vi "Capture@FeatureMatchOne__Parameter.vi"(1 "ParamterIn":string) -> (0 "ParamterOut":string)   [LabVIEW 2020]
uses:
  MainFrame/Global.vi
panel:
  out "Image":T1(plugin-control)
  in  "Picture":string(combo)
  in  "AngleEnd":string(combo)
  in  "AngleStart":string(combo)
  in  "Score":string(combo)="50"
  in  "Point":string(combo)
  in  "CamName":string(combo)
  in  "Confirm":bool
  # "Capture@FeatureMatchOne $Capture,$Picture,$Score,$Point(,$Angle=XX~XX)"
  # "Angle="
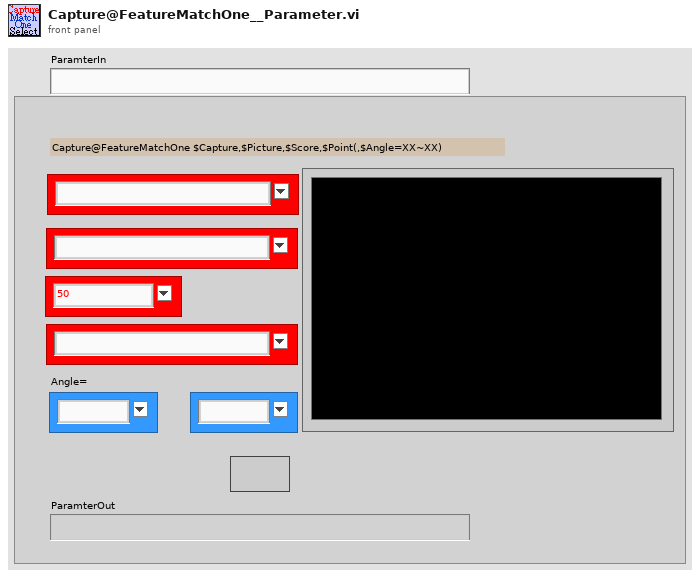
[diagram p1: front panel]
types:
  T1 = typedef "IMAQ Image.ctl" = refnum<image>
  T2 = enum16{"Get", "UpdatePointS", "Init", "UpdateIndex", "GetCurrent&Index+1", "GetWithIndex", "ChkLast", "GetCurrent"}
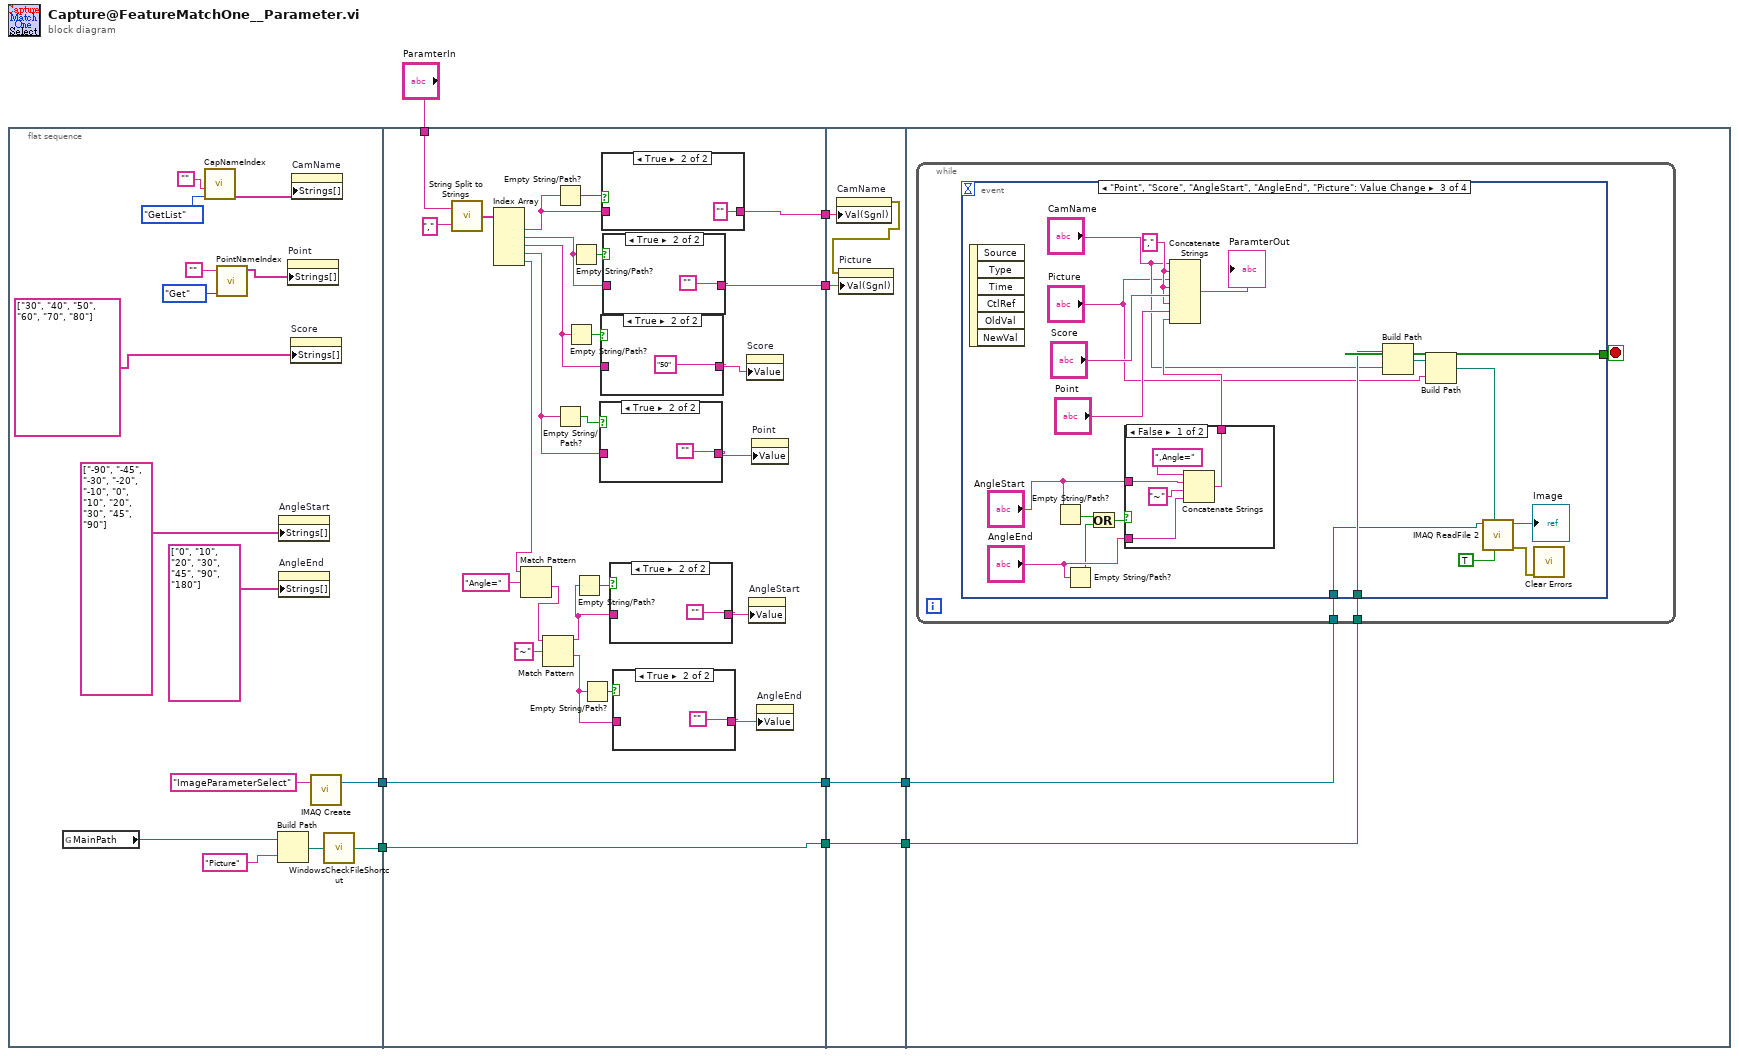
[diagram p0: block diagram]
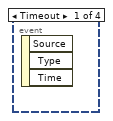
[diagram p8: hidden frame]
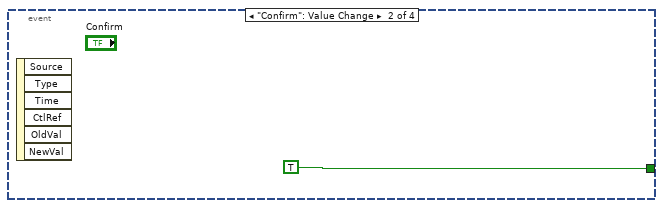
[diagram p9: hidden frame]
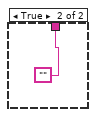
[diagram p10: hidden frame]
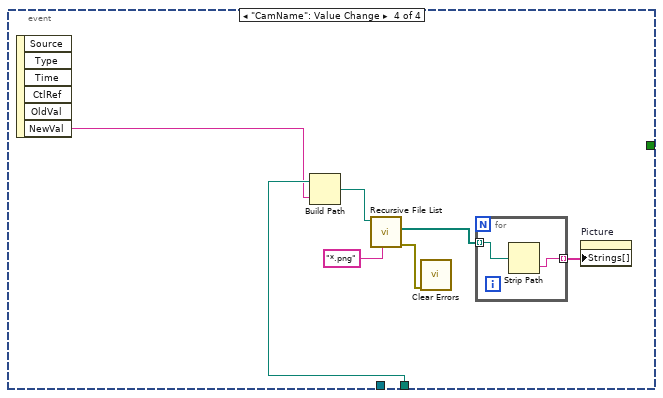
[diagram p11: hidden frame]
diagram:
  n1 = flat-sequence {
    tunnel: [w16] -> w8
    tunnel: [w10] -> w3
    tunnel: "ParamterIn" -> [w49]
    tunnel: w8 -> [w30]
    tunnel: [w30] -> w7
    tunnel: [w28] -> w4
    tunnel: w3 -> [w28]
    tunnel: [w26] -> w2
    tunnel: [w25] -> w1
    tunnel: w7 -> [w68]
    tunnel: [w68] -> w6
    tunnel: [w67] -> w5
    tunnel: w4 -> [w67]
    tunnel: w2 -> [w66]
    tunnel: w1 -> [w65]
    tunnel: w6 -> [w70]
    tunnel: w5 -> [w69]
    frame #0 {
      n2 = global read "Global.vi" "MainPath"() -> (w13:path)
      n3 = call "CapNameIndex.vi"("OP"=enum16{"AddCam", "GetIndex", "Init", "GetList"}."GetList", "CamName"="") -> ("DeviceList"=w23:string[])  [unwired: 2 in, 3 out]
      n4 = call "PointNameIndex.vi"("OP"=T2."Get", "PointName"="") -> ("PointNameList"=w19:string[])  [unwired: 4 in, 5 out]
      n5 = Build Path(base path=w13, name or relative path="Picture") -> (appended path=w11:path)
      n6 = property on="AngleStart" class="CmbBox"("Strings[]"=string[] ["-90", "-45", "-30", "-20", "-10", "0", "10", "20", "30", "45", "90"] ("Strings []")) -> ()  [unwired: 2 in, 2 out]
      n7 = property on="AngleEnd" class="CmbBox"("Strings[]"=string[] ["0", "10", "20", "30", "45", "90", "180"] ("Strings []")) -> ()  [unwired: 2 in, 2 out]
      n8 = property on="Point" class="CmbBox"("Strings[]"=w19) -> ()  [unwired: 2 in, 2 out]
      n9 = property on="Score" class="CmbBox"("Strings[]"=string[] ["30", "40", "50", "60", "70", "80"] ("Strings []")) -> ()  [unwired: 2 in, 2 out]
      n10 = property on="CamName" class="CmbBox"("Strings[]"=w23) -> ()  [unwired: 2 in, 2 out]
      n11 = call "IMAQ Create"("Image Name"="ImageParameterSelect") -> ("New Image"=w16:T1)  [unwired: 4 in, 1 out]
      n12 = call "WindowsCheckFileShortcut.vi"("LinkPath"=w11) -> ("TargetPath"=w10:path)  [unwired: 4 in]
    }
    frame #1 {
      n13 = call "String Split to Strings.vi"("search string/char (-)"=",", "String"=w49) -> ("Array"=w51:string[])
      n14 = Index Array(array=w51) -> (element #1=w29:string, element #2=w41:string, element #3=w44:string, element #4=w46:string, element #5=w40:string)  [unwired: 5 in]
      n15 = Match Pattern(string=w40, regular expression="Angle=") -> (after substring=w38:string)  [unwired: 1 in, 3 out]
      n16 = Match Pattern(string=w38, regular expression="~") -> (before substring=w35:string, after substring=w33:string)  [unwired: 1 in, 2 out]
      n17 = Empty String/Path?(string/path=w29) -> (empty?=w48:bool)
      n18 = Empty String/Path?(string/path=w46) -> (empty?=w47:bool)
      n19 = Empty String/Path?(string/path=w44) -> (empty?=w45:bool)
      n20 = Empty String/Path?(string/path=w41) -> (empty?=w42:bool)
      n21 = Empty String/Path?(string/path=w35) -> (empty?=w36:bool)
      n22 = Empty String/Path?(string/path=w33) -> (empty?=w34:bool)
      n23 = case shown="True" w47 {
        tunnel: [w60 ""] -> w27
        tunnel: w46 -> [w60 _]
        frame False {
        }
        frame True {
        }
      }
      n24 = case shown="True" w45 {
        tunnel: [w58 "50"] -> w43
        tunnel: w44 -> [w58 _]
        frame False {
        }
        frame True {
        }
      }
      n25 = case shown="True" w48 {
        tunnel: w29 -> [w62 _]
        tunnel: [w62 ""] -> w25
        frame False {
        }
        frame True {
        }
      }
      n26 = case shown="True" w42 {
        tunnel: [w56 ""] -> w26
        tunnel: w41 -> [w56 _]
        frame False {
        }
        frame True {
        }
      }
      n27 = case shown="True" w36 {
        tunnel: [w54 ""] -> w32
        tunnel: w35 -> [w54 _]
        frame False {
        }
        frame True {
        }
      }
      n28 = case shown="True" w34 {
        tunnel: [w52 ""] -> w31
        tunnel: w33 -> [w52 _]
        frame False {
        }
        frame True {
        }
      }
      n29 = property on="Score" class="CmbBox"("Value"=w43) -> ()  [unwired: 2 in, 2 out]
      n30 = property on="AngleStart" class="CmbBox"("Value"=w32) -> ()  [unwired: 2 in, 2 out]
      n31 = property on="Point" class="CmbBox"("Value"=w27) -> ()  [unwired: 2 in, 2 out]
      n32 = property on="AngleEnd" class="CmbBox"("Value"=w31) -> ()  [unwired: 2 in, 2 out]
    }
    frame #2 {
      n33 = property on="CamName" class="CmbBox"("Val(Sgnl)"=w65) -> (error out=w64:errorcluster)  [unwired: 2 in, 1 out]
      n34 = property on="Picture" class="CmbBox"(error in=w64, "Val(Sgnl)"=w66) -> ()  [unwired: 1 in, 2 out]
    }
    frame #3 {
      n35 = while {
        tunnel: w70 -> [w72]
        tunnel: w69 -> [w71]
        stop <- w73 stop-if-true
        n36 = event shown="[2] \"Point\", \"Score\", \"AngleStart\", \"AngleEnd\", \"Picture\": Value Change" {
          selector: _ -> [_ _ _ _]
          dyn-events: _ -> [_ _ _ _]
          timeout: _ -> [_ _ _ _]
          tunnel: [_ TRUE _ _] -> w73
          tunnel: w72 -> [_ _ w76 _]
          tunnel: w71 -> [_ _ w83 w103]
          event Timeout {
            n37 = event-data() -> ()  [unwired: 1 in, 3 out]
          }
          event "Confirm": Value Change {
            n38 = event-data() -> ()  [unwired: 1 in, 6 out]
          }
          event "Point", "Score", "AngleStart", "AngleEnd", "Picture": Value Change {
            w90 = "," ("string")
            n39 = event-data() -> ()  [unwired: 1 in, 6 out]
            n40 = Empty String/Path?(string/path="AngleStart") -> (empty?=w85:bool)
            n41 = Empty String/Path?(string/path="AngleEnd") -> (empty?=w84:bool)
            n42 = Or(x=w85, y=w84) -> (x .or. y?=w86:bool)
            n43 = case shown="False" w86 {
              tunnel: [w96 ""] -> w89
              tunnel: "AngleStart" -> [w95 _]
              tunnel: "AngleEnd" -> [w94 _]
              frame False {
                n44 = Concatenate Strings(",Angle=" ("string"), w95, "~", w94) -> (w96:string)
              }
              frame True {
              }
            }
            n45 = Concatenate Strings("CamName", w90, "Picture", w90, "Score", w90, "Point", w89) -> (→"ParamterOut":string)
            n46 = Build Path(base path=w83, name or relative path="CamName") -> (appended path=w81:path)
            n47 = Build Path(base path=w81, name or relative path="Picture") -> (appended path=w79:path)
            n48 = call "IMAQ ReadFile 2"("Use File Path Image Type"=TRUE, "File Path"=w79, "Image"=w76) -> ("error out"=w78:errorcluster, "Image Out"=→"Image":T1)  [unwired: 4 in, 3 out]
            n49 = call <vilib>:"Clear Errors.vi"("error in (no error)"=w78) -> ()  [unwired: 5 in, 2 out]
          }
          event "CamName": Value Change {
            n50 = event-data() -> ("NewVal"=w102:string)  [unwired: 1 in, 5 out]
            n51 = Build Path(base path=w103, name or relative path=w102) -> (appended path=w101:path)
            n52 = call <vilib>:"Recursive File List.vi"("pattern"="*.png", "Folder Path"=w101) -> ("error out"=w100:errorcluster, "All Files in Dir"=w105:path[])  [unwired: 5 in, 3 out]
            n53 = call <vilib>:"Clear Errors.vi"("error in (no error)"=w100) -> ()  [unwired: 5 in, 2 out]
            n54 = for {
              tunnel: w105 -> [w108] mode=indexing
              tunnel: [w107] -> w106 mode=indexing
              n55 = Strip Path(path=w108) -> (name=w107:string)  [unwired: 1 out]
            }
            n56 = property on="Picture" class="CmbBox"("Strings[]"=w106) -> ()  [unwired: 2 in, 2 out]
          }
        }
      }
    }
  }
